vi "Manage Dialog.vi"() -> ()   [LabVIEW 2011, in "CAN FD.lvlib"]
uses:
  CAN FD.lvlib
  Typedef/ManUIref.ctl
panel:
  in  "Close":bool
  in  "2Ch1Stop":bool
  in  "2Ch1Start":bool
  out "Ch1":string
  in  "1Ch0Stop":bool
  in  "1Ch0Start":bool
  out "Ch0":string
  in  "0DevStop":bool
  in  "0DevStart":bool
  out "Device":string
  in  "DevInfo":bool
  in  "Open":bool
  in  "Index":u32(ring) caption="索引" items=["0", "1", "2", "3", "4", "5", "6", "7", "8"]
  in  "Type":u32(ring)=41 caption="CAN卡型号" items=["USBCANFD"=41]
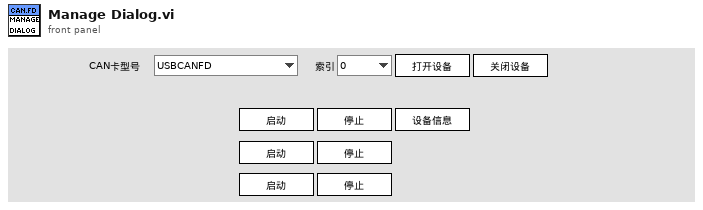
[diagram p1: front panel]
types:
  T1 = typedef "CAN FD.lvlib/ManUIref.ctl" = cluster{"Type":refnum<vi>, "Index":refnum<vi>, "Open":refnum<vi>, "Close":refnum<vi>, "Device":refnum<vi>, "DevStart":refnum<vi>, "DevStop":refnum<vi>, "DevInfo":refnum<vi>, "Ch0":refnum<vi>, "Ch0Start":refnum<vi>, "Ch0Stop":refnum<vi>, "Ch1":refnum<vi>, "Ch1Start":refnum<vi>, "Ch1Stop":refnum<vi>}
  T2 = cluster{"Type":u32, "Index":u32, "DeviceOpen":bool, "Ch0Start":bool, "Ch1Start":bool}
  T3 = cluster{"hw_ver":dbl, "fw_ver":dbl, "dr_ver":dbl, "in_ver":dbl, "irq_Num":u16, "can_Num":u8, "SN":string, "hw_type":string}
  T4 = cluster{"Enable":bool, "Config":cluster{"Mode":enum16{"标准帧组ID", "标准帧明确ID", "扩展帧组ID", "扩展帧明确ID"}, "Start":u32, "End":u32}[]}
  T5 = cluster{"Terminal":u32, "Param":cluster{"abitbaud":u32, "dbitbaud":u32, "CustomBaud":bool, "CustomBd":string, "Mode":u8, "Standard":u32}}
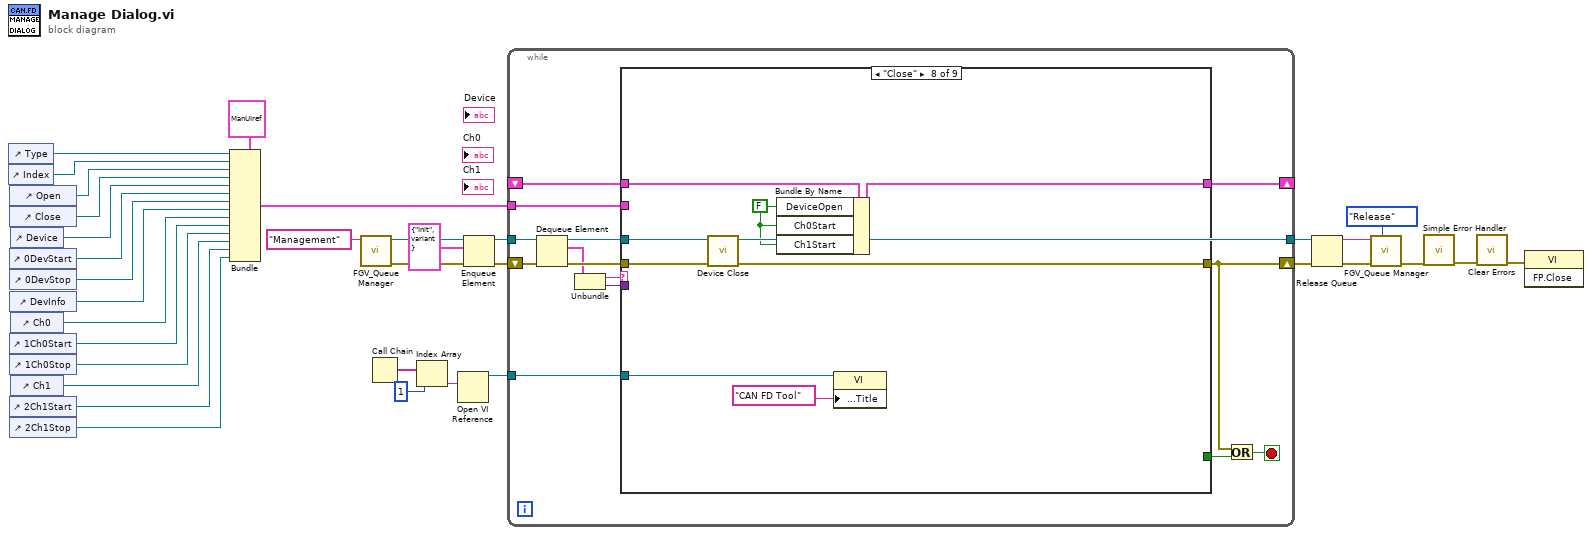
[diagram p0: block diagram]
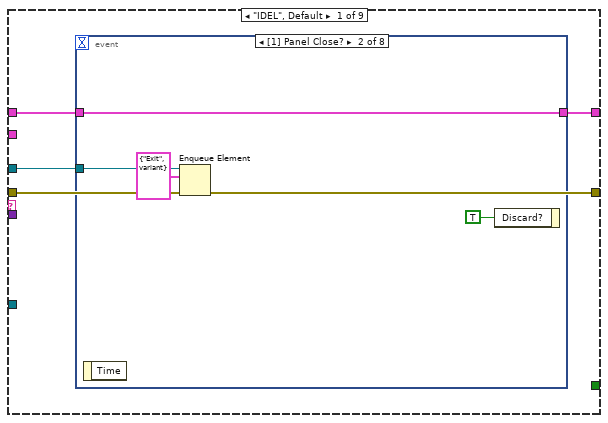
[diagram p2: hidden frame]
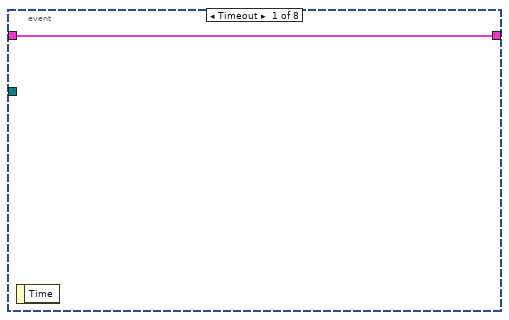
[diagram p3: hidden frame]
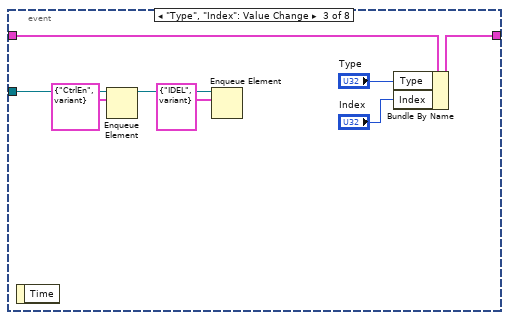
[diagram p4: hidden frame]
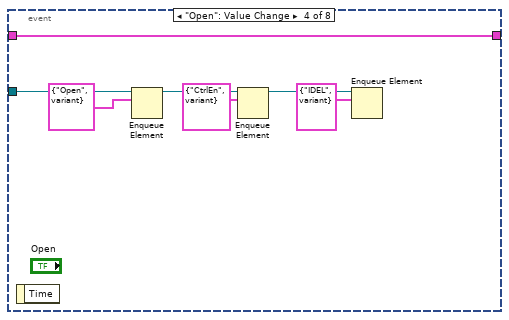
[diagram p5: hidden frame]
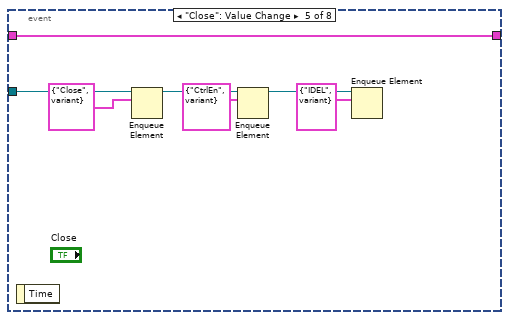
[diagram p6: hidden frame]
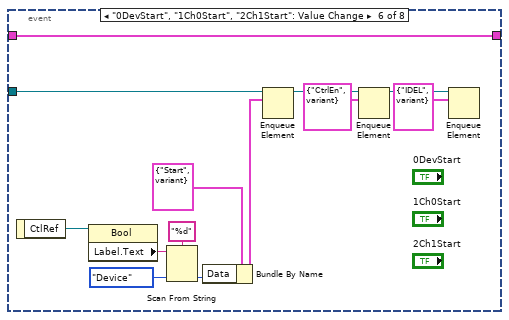
[diagram p7: hidden frame]
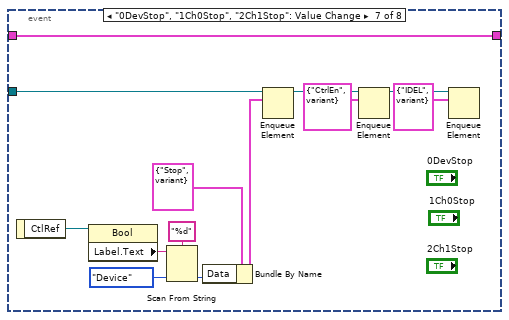
[diagram p8: hidden frame]
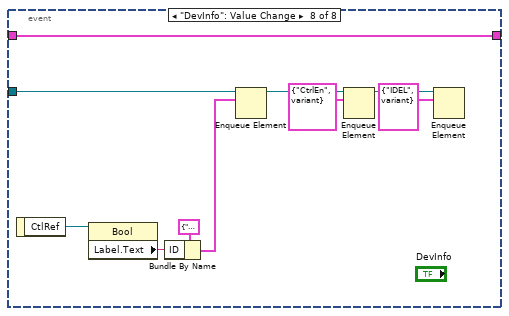
[diagram p9: hidden frame]
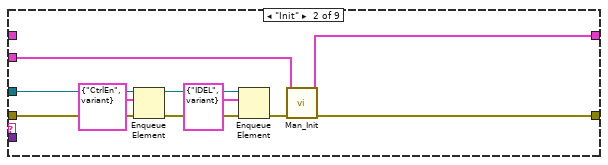
[diagram p10: hidden frame]
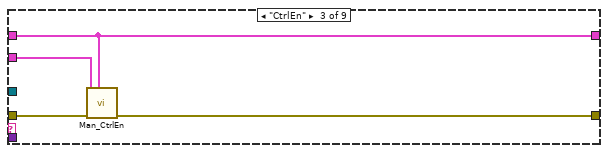
[diagram p11: hidden frame]
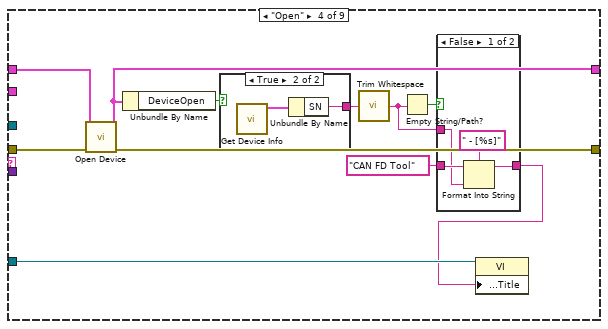
[diagram p12: hidden frame]
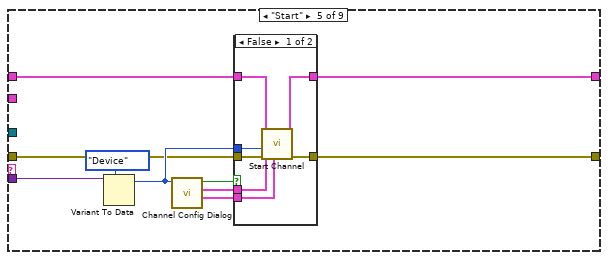
[diagram p15: hidden frame]
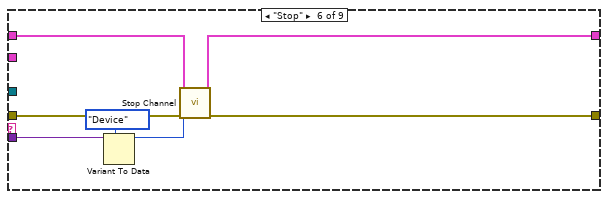
[diagram p17: hidden frame]
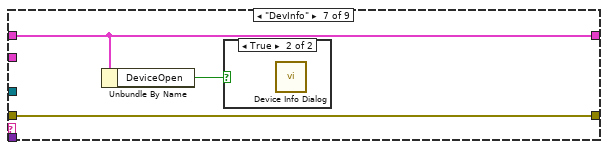
[diagram p18: hidden frame]
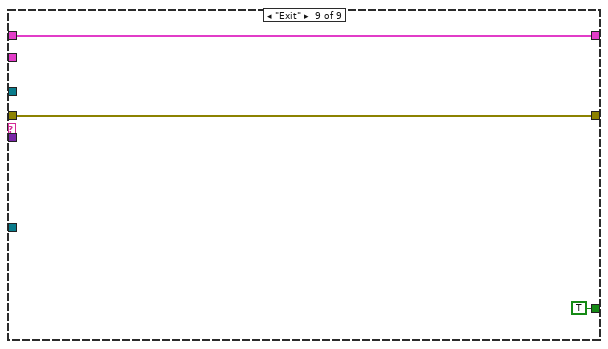
[diagram p20: hidden frame]
diagram:
  n1 = control-ref of="Type"() -> (w24:refnum<vi>)
  n2 = control-ref of="Index"() -> (w23:refnum<vi>)
  n3 = control-ref of="Open"() -> (w22:refnum<vi>)
  n4 = control-ref of="Close"() -> (w21:refnum<vi>)
  n5 = control-ref of="0DevStart"() -> (w19:refnum<vi>)
  n6 = control-ref of="0DevStop"() -> (w18:refnum<vi>)
  n7 = control-ref of="DevInfo"() -> (w17:refnum<vi>)
  n8 = control-ref of="1Ch0Start"() -> (w15:refnum<vi>)
  n9 = control-ref of="1Ch0Stop"() -> (w14:refnum<vi>)
  n10 = control-ref of="2Ch1Start"() -> (w12:refnum<vi>)
  n11 = control-ref of="2Ch1Stop"() -> (w11:refnum<vi>)
  n12 = control-ref of="Device"() -> (w20:refnum<vi>)
  n13 = control-ref of="Ch0"() -> (w16:refnum<vi>)
  n14 = control-ref of="Ch1"() -> (w13:refnum<vi>)
  n15 = Bundle(cluster=T1 {"Type"=refnum, "Index"=refnum, "Open"=refnum, "Close"=refnum, "Device"=refnum, "DevStart"=refnum, "DevStop"=refnum, "DevInfo"=refnum, "Ch0"=refnum, "Ch0Start"=refnum, "Ch0Stop"=refnum, "Ch1"=refnum, "Ch1Start"=refnum, "Ch1Stop"=refnum} ("ManUIref"), "Type"=w24, "Index"=w23, "Open"=w22, "Close"=w21, "Device"=w20, "DevStart"=w19, "DevStop"=w18, "DevInfo"=w17, "Ch0"=w16, "Ch0Start"=w15, "Ch0Stop"=w14, "Ch1"=w13, "Ch1Start"=w12, "Ch1Stop"=w11) -> (w9:T1)
  n16 = call "FGV_Queue Manager.vi"("Name"="Management") -> ("error out"=w33:errorcluster, "Queue"=w34:refnum<queue>)  [unwired: 8 in, 1 out]
  n17 = Call Chain() -> (call chain=w4:string[])
  n18 = Index Array(array=w4, index=1) -> (element=w2:string)
  n19 = Open VI Reference(vi path=w2) -> (vi reference=w1:refnum<vi>)  [unwired: 5 in, 1 out]
  n20 = Enqueue Element(queue=w34, element=cluster{"ID":string, "Data":variant} {"ID"="Init", "Data"=variant} ("元素"), error in (no error)=w33) -> (queue out=w29:refnum<queue>, error out=w30:errorcluster)  [unwired: 1 in, 1 out]
  n21 = while {
    tunnel: w29 -> [w47]
    tunnel: [w38] -> w27
    shift-right: [w39] -> w28
    shift-left: w30 -> [w48]
    tunnel: w9 -> [w40]
    shift-right: [w37] -> _
    shift-left: _ -> [w36]
    tunnel: w1 -> [w35]
    stop <- w42 stop-if-true
    n22 = Dequeue Element(queue=w47, error in (no error)=w48) -> (queue out=w38:refnum<queue>, element=w41:cluster{"ID":string, "Data":variant}, error out=w44:errorcluster)  [unwired: 1 in, 1 out]
    n23 = Unbundle(w41) -> ("ID"=w46:string, "Data"=w45:variant)
    n24 = case shown="\"Close\"" w46 {
      tunnel: w45 -> [_ _ _ _ w157 w173 _ _ _]
      tunnel: [_ _ _ _ _ _ _ _ TRUE] -> w43
      tunnel: [w52 w123 w128 w139 w149 w170 w176 w182 w185] -> w39
      tunnel: w44 -> [w52 w118 w129 w140 w150 w171 w176 w183 w185]
      tunnel: w38 -> [w51 w119 _ _ _ _ _ _ _]
      tunnel: w40 -> [_ w121 w127 _ _ _ _ _ _]
      tunnel: [w50 w122 w126 w137 w152 w168 w175 w179 w184] -> w37
      tunnel: w36 -> [w49 _ w126 w138 w151 w169 w175 w181 w184]
      tunnel: w35 -> [_ _ _ w131 _ _ _ w177 _]
      frame "IDEL", Default {
        n25 = event shown="[1] Panel Close?" {
          selector: _ -> [_ _ _ _ _ _ _ _]
          dyn-events: _ -> [_ _ _ _ _ _ _ _]
          timeout: _ -> [_ _ _ _ _ _ _ _]
          tunnel: w51 -> [_ w56 w62 w70 w77 w90 w103 w108]
          tunnel: [w53 w54 w58 w72 w79 w92 w105 w115] -> w50
          tunnel: w49 -> [w53 w54 w61 w72 w79 w92 w105 w115]
          event Timeout {
            n26 = event-data() -> ()  [unwired: 1 in, 1 out]
          }
          event Panel Close? {
            n27 = event-data() -> ()  [unwired: 1 in, 1 out]
            n28 = Enqueue Element(queue=w56, element=cluster{"ID":string, "Data":variant} {"ID"="Exit", "Data"=variant} ("元素")) -> ()  [unwired: 2 in, 3 out]
            n29 = event-data("Discard?"=TRUE ("放弃？")) -> ()  [unwired: 1 in, 1 out]
          }
          event "Type", "Index": Value Change {
            n30 = event-data() -> ()  [unwired: 1 in, 1 out]
            n31 = Enqueue Element(queue=w62, element=cluster{"ID":string, "Data":variant} {"ID"="CtrlEn", "Data"=variant} ("元素")) -> (queue out=w63:refnum<queue>)  [unwired: 2 in, 2 out]
            n32 = Enqueue Element(queue=w63, element=cluster{"ID":string, "Data":variant} {"ID"="IDEL", "Data"=variant} ("元素")) -> ()  [unwired: 2 in, 3 out]
            n33 = Bundle By Name(cluster=w61, "Type"="Type", "Index"="Index") -> (w58:T2)
          }
          event "Open": Value Change {
            n34 = event-data() -> ()  [unwired: 1 in, 1 out]
            n35 = Enqueue Element(queue=w70, element=cluster{"ID":string, "Data":variant} {"ID"="Open", "Data"=variant} ("元素")) -> (queue out=w67:refnum<queue>)  [unwired: 2 in, 2 out]
            n36 = Enqueue Element(queue=w67, element=cluster{"ID":string, "Data":variant} {"ID"="CtrlEn", "Data"=variant} ("元素")) -> (queue out=w66:refnum<queue>)  [unwired: 2 in, 2 out]
            n37 = Enqueue Element(queue=w66, element=cluster{"ID":string, "Data":variant} {"ID"="IDEL", "Data"=variant} ("元素")) -> ()  [unwired: 2 in, 3 out]
          }
          event "Close": Value Change {
            n38 = event-data() -> ()  [unwired: 1 in, 1 out]
            n39 = Enqueue Element(queue=w77, element=cluster{"ID":string, "Data":variant} {"ID"="Close", "Data"=variant} ("元素")) -> (queue out=w74:refnum<queue>)  [unwired: 2 in, 2 out]
            n40 = Enqueue Element(queue=w74, element=cluster{"ID":string, "Data":variant} {"ID"="CtrlEn", "Data"=variant} ("元素")) -> (queue out=w73:refnum<queue>)  [unwired: 2 in, 2 out]
            n41 = Enqueue Element(queue=w73, element=cluster{"ID":string, "Data":variant} {"ID"="IDEL", "Data"=variant} ("元素")) -> ()  [unwired: 2 in, 3 out]
          }
          event "0DevStart", "1Ch0Start", "2Ch1Start": Value Change {
            n42 = event-data() -> ("CtlRef"=w84:refnum<vi>)  [unwired: 1 in]
            n43 = property class="Bool"(reference=w84) -> ("Label.Text"=w82:string)  [unwired: 1 in, 2 out]
            n44 = Scan From String(format string="%d" ("格式字符串"), input string=w82, default 1=enum16{"Device", "Ch0", "Ch1"}."Device") -> (output 1=w80:enum16{"Device", "Ch0", "Ch1"})  [unwired: 2 in, 3 out]
            n45 = Bundle By Name(cluster=cluster{"ID":string, "Data":variant} {"ID"="Start", "Data"=variant} ("元素"), "Data"=w80) -> (w85:cluster{"ID":string, "Data":variant})
            n46 = Enqueue Element(queue=w90, element=w85) -> (queue out=w88:refnum<queue>)  [unwired: 2 in, 2 out]
            n47 = Enqueue Element(queue=w88, element=cluster{"ID":string, "Data":variant} {"ID"="CtrlEn", "Data"=variant} ("元素")) -> (queue out=w87:refnum<queue>)  [unwired: 2 in, 2 out]
            n48 = Enqueue Element(queue=w87, element=cluster{"ID":string, "Data":variant} {"ID"="IDEL", "Data"=variant} ("元素")) -> ()  [unwired: 2 in, 3 out]
          }
          event "0DevStop", "1Ch0Stop", "2Ch1Stop": Value Change {
            n49 = event-data() -> ("CtlRef"=w97:refnum<vi>)  [unwired: 1 in]
            n50 = property class="Bool"(reference=w97) -> ("Label.Text"=w95:string)  [unwired: 1 in, 2 out]
            n51 = Scan From String(format string="%d" ("格式字符串"), input string=w95, default 1=enum16{"Device", "Ch0", "Ch1"}."Device") -> (output 1=w93:enum16{"Device", "Ch0", "Ch1"})  [unwired: 2 in, 3 out]
            n52 = Bundle By Name(cluster=cluster{"ID":string, "Data":variant} {"ID"="Stop", "Data"=variant} ("元素"), "Data"=w93) -> (w98:cluster{"ID":string, "Data":variant})
            n53 = Enqueue Element(queue=w103, element=w98) -> (queue out=w101:refnum<queue>)  [unwired: 2 in, 2 out]
            n54 = Enqueue Element(queue=w101, element=cluster{"ID":string, "Data":variant} {"ID"="CtrlEn", "Data"=variant} ("元素")) -> (queue out=w100:refnum<queue>)  [unwired: 2 in, 2 out]
            n55 = Enqueue Element(queue=w100, element=cluster{"ID":string, "Data":variant} {"ID"="IDEL", "Data"=variant} ("元素")) -> ()  [unwired: 2 in, 3 out]
          }
          event "DevInfo": Value Change {
            n56 = event-data() -> ("CtlRef"=w111:refnum<vi>)  [unwired: 1 in]
            n57 = property class="Bool"(reference=w111) -> ("Label.Text"=w109:string)  [unwired: 1 in, 2 out]
            n58 = Bundle By Name(cluster=cluster{"ID":string, "Data":variant} {"ID"="", "Data"=variant} ("元素"), "ID"=w109) -> (w106:cluster{"ID":string, "Data":variant})
            n59 = Enqueue Element(queue=w108, element=w106) -> (queue out=w107:refnum<queue>)  [unwired: 2 in, 2 out]
            n60 = Enqueue Element(queue=w107, element=cluster{"ID":string, "Data":variant} {"ID"="CtrlEn", "Data"=variant} ("元素")) -> (queue out=w112:refnum<queue>)  [unwired: 2 in, 2 out]
            n61 = Enqueue Element(queue=w112, element=cluster{"ID":string, "Data":variant} {"ID"="IDEL", "Data"=variant} ("元素")) -> ()  [unwired: 2 in, 3 out]
          }
        }
      }
      frame "Init" {
        n62 = Enqueue Element(queue=w119, element=cluster{"ID":string, "Data":variant} {"ID"="CtrlEn", "Data"=variant} ("元素"), error in (no error)=w118) -> (queue out=w117:refnum<queue>, error out=w116:errorcluster)  [unwired: 1 in, 1 out]
        n63 = Enqueue Element(queue=w117, element=cluster{"ID":string, "Data":variant} {"ID"="IDEL", "Data"=variant} ("元素"), error in (no error)=w116) -> (error out=w124:errorcluster)  [unwired: 1 in, 2 out]
        n64 = call "Man_Init.vi"("error in (no error)"=w124, "ManUIref"=w121) -> ("error out"=w123:errorcluster, "DevState"=w122:T2)  [unwired: 8 in]
      }
      frame "CtrlEn" {
        n65 = call "Man_CtrlEn.vi"("DevState"=w126, "error in (no error)"=w129, "ManUIref"=w127) -> ("error out"=w128:errorcluster)  [unwired: 8 in]
      }
      frame "Open" {
        n66 = call "Open Device.vi"("error in (no error)"=w140, "DevState"=w138) -> ("error out"=w139:errorcluster, "DevState out"=w137:T2)  [unwired: 8 in]
        n67 = Unbundle By Name(w137) -> ("DeviceOpen"=w136:bool)
        n68 = case shown="True" w136 {
          tunnel: [_ w146] -> w135
          frame False {
          }
          frame True {
            n69 = call "Get Device Info.vi"() -> ("device info"=w147:T3)  [unwired: 9 in, 2 out]
            n70 = Unbundle By Name(w147) -> ("SN"=w146:string)
          }
        }
        n71 = call <vilib>:"Trim Whitespace.vi"("string"=w135) -> ("trimmed string"=w133:string)  [unwired: 1 in]
        n72 = Empty String/Path?(string/path=w133) -> (empty?=w134:bool)
        n73 = case shown="False" w134 {
          tunnel: w133 -> [w142 _]
          tunnel: "CAN FD Tool" -> [w143 w145]
          tunnel: [w144 w145] -> w130
          frame False {
            n74 = Format Into String(format string=" - [%s]", initial string=w143, w142) -> (resulting string=w144:string)  [unwired: 1 in, 1 out]
          }
          frame True {
          }
        }
        n75 = property class="VI"(reference=w131, "Front Panel.Title"=w130) -> ()  [unwired: 1 in, 2 out]
      }
      frame "Start" {
        n76 = Variant To Data(type=enum16{"Device", "Ch0", "Ch1"}."Device", Variant=w157) -> (data=w153:enum16{"Device", "Ch0", "Ch1"})  [unwired: 1 in, 1 out]
        n77 = call "Channel Config Dialog.vi"("Type"=w153) -> ("Filter"=w148:T4, "Param"=w154:T5, "Cancel"=w155:bool)  [unwired: 7 in, 1 out]
        n78 = case shown="False" w155 {
          tunnel: w154 -> [w159 _]
          tunnel: w153 -> [w160 _]
          tunnel: [w161 w166] -> w152
          tunnel: w151 -> [w162 w166]
          tunnel: w150 -> [w164 w165]
          tunnel: [w163 w165] -> w149
          tunnel: w148 -> [w158 _]
          frame False {
            n79 = call "Start Channel.vi"("Filter"=w158, "error in (no error)"=w164, "ChannelType"=w160, "Param"=w159, "DevState"=w162) -> ("error out"=w163:errorcluster, "DevState out"=w161:T2)  [unwired: 5 in]
          }
          frame True {
          }
        }
      }
      frame "Stop" {
        n80 = Variant To Data(type=enum16{"Device", "Ch0", "Ch1"}."Device", Variant=w173) -> (data=w167:enum16{"Device", "Ch0", "Ch1"})  [unwired: 1 in, 1 out]
        n81 = call "Stop Channel.vi"("error in (no error)"=w171, "ChannelType"=w167, "DevState"=w169) -> ("error out"=w170:errorcluster, "DevState out"=w168:T2)  [unwired: 7 in]
      }
      frame "DevInfo" {
        n82 = Unbundle By Name(w175) -> ("DeviceOpen"=w174:bool)
        n83 = case shown="True" w174 {
          frame False {
          }
          frame True {
            n84 = call "Device Info Dialog.vi"() -> ()  [unwired: 12 in]
          }
        }
      }
      frame "Close" {
        w180 = FALSE ("DeviceOpen")
        n85 = call "Device Close.vi"("error in (no error)"=w183) -> ("error out"=w182:errorcluster)  [unwired: 10 in]
        n86 = Bundle By Name(cluster=w181, "DeviceOpen"=w180, "Ch0Start"=w180, "Ch1Start"=w180) -> (w179:T2)
        n87 = property class="VI"(reference=w177, "Front Panel.Title"="CAN FD Tool") -> ()  [unwired: 1 in, 2 out]
      }
      frame "Exit" {
      }
    }
    n88 = Or(x=w39, y=w43) -> (x .or. y?=w42:bool)
  }
  n89 = Release Queue(queue=w27, error in (no error)=w28) -> (queue name=w7:string, error out=w8:errorcluster)  [unwired: 1 in, 1 out]
  n90 = call "FGV_Queue Manager.vi"("Methods"=enum16{"Init", "Get", "Release", "Destroy"}."Release", "error in (no error)"=w8, "Name"=w7) -> ("error out"=w6:errorcluster)  [unwired: 6 in, 2 out]
  n91 = call <vilib>:"Simple Error Handler.vi"("error in (no error)"=w6) -> ("error out"=w26:errorcluster)  [unwired: 4 in, 4 out]
  n92 = call <vilib>:"Clear Errors.vi"("error in (no error)"=w26) -> ("error out"=w25:errorcluster)  [unwired: 6 in]
  n93 = invoke class="VI" method="FP.Close"(error in=w25) -> ()  [unwired: 2 in, 3 out]
